vi "Read Registry Value Simple.vi"   [LabVIEW 2012]
doc: "Reads data and the simplified data type from a registry value. If the key or value does not exist or an unrecoverable error occurs, the VI returns the default data. Wire data to the <B>default data</B> input to determine the polymorphic instance to use or manually select the instance."
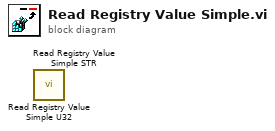
[diagram p0: block diagram]
diagram:
  n1 = call "Read Registry Value Simple U32.vi"() -> ()  [unwired: 6 in, 4 out]
  n2 = call "Read Registry Value Simple STR.vi"() -> ()  [unwired: 6 in, 4 out]
